vi "_dll_path.vi"() -> (1 "Path":path)   [LabVIEW 2019, in "gfitsio.lvlib"]
uses:
  gfitsio.lvlib
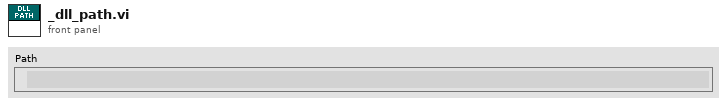
[diagram p1: front panel]
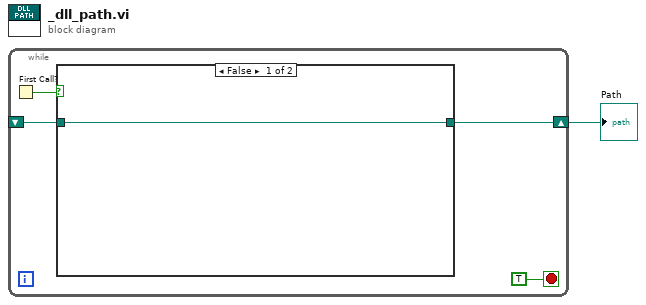
[diagram p0: block diagram]
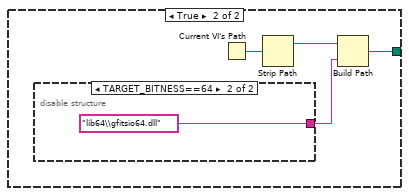
[diagram p2: hidden frame]
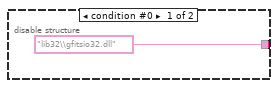
[diagram p3: hidden frame]
diagram:
  n1 = while {
    shift-right: [w5] -> w1
    shift-left: _ -> [w2]
    stop <- TRUE stop-if-true
    n2 = First Call?() -> (First Call?: T/F=w3:bool)
    n3 = case shown="False" w3 {
      tunnel: [w6 w7] -> w5
      tunnel: w2 -> [w6 _]
      frame False {
      }
      frame True {
        n4 = disable-structure shown="TARGET_BITNESS==64" {
          disable-tunnel: ["lib32\\gfitsio32.dll" ("name or relative path") "lib64\\gfitsio64.dll" ("name or relative path")] -> w8
          frame condition #0 {
          }
          frame condition #1 (active) {
          }
        }
        n5 = Current VI's Path() -> (path=w9:path)
        n6 = Strip Path(path=w9) -> (stripped path=w10:path)  [unwired: 1 out]
        n7 = Build Path(base path=w10, name or relative path=w8) -> (appended path=w7:path)
      }
    }
  }
  "Path" <- w1
